vi "CS POLARIS BME DG.write changes to file.vi"(7 "error in":errorcluster, 9 "BME_DG_System in":refnum<class "BME_DG_System.lvclass">, 10 "i ref in":refnum<vi>) -> (0 "error in":errorcluster, 2 "BME_DG_System out":refnum<class "BME_DG_System.lvclass">, 3 "i ref out":refnum<vi>)   [LabVIEW 2009, in "CS POLARIS BME DG.lvlib"]
uses:
  CS POLARIS BME DG.lvlib
  DG Classes/BME_DG_System/BME_DG_System.lvclass
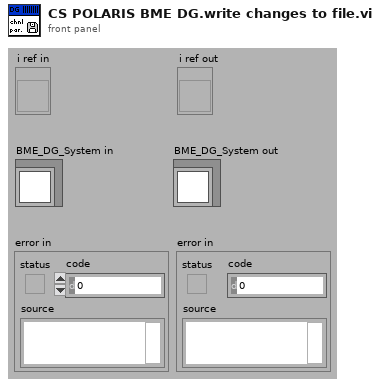
[diagram p1: front panel]
types:
  T1 = typedef "CS POLARIS BME DG.lvlib/CS POLARIS BME DG.i attribute.ctl" = cluster{"DIMLockedBy":i32, "DG_System":refnum<queue>, "UpdateTasks":refnum<queue>, "SaveEachParamChng":bool, "SaveAtShutdown":bool}
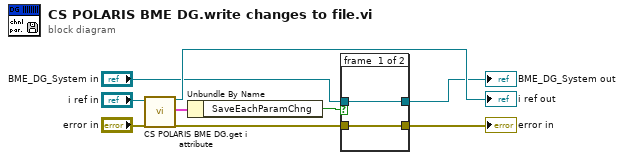
[diagram p0: block diagram]
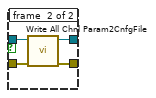
[diagram p2: hidden frame]
diagram:
  n1 = call "CS POLARIS BME DG.get i attribute.vi"("i ref in"="i ref in", "error in (no error)"="error in") -> ("i ref out"=→"i ref out":refnum<vi>, "i attribute"=w7:T1, "error out"=w5:errorcluster)  [unwired: 15 in]
  n2 = Unbundle By Name(w7) -> ("SaveEachParamChng"=w2:bool)
  n3 = case shown="True" w2 {
    tunnel: w5 -> [w10 w15]
    tunnel: "BME_DG_System in" -> [w11 w14]
    tunnel: [w10 w13] -> w3
    tunnel: [w11 w12] -> w1
    frame #0 {
    }
    frame #1 {
      n4 = call "Write All Chnl Param2CnfgFile.vi"("error in (no error)"=w15, "BME_DG_System in"=w14) -> ("error out"=w13:errorcluster, "BME_DG_System out"=w12:refnum<class "BME_DG_System.lvclass">)  [unwired: 8 in]
    }
  }
  "error in" <- w3
  "BME_DG_System out" <- w1
